vi "Apply Scaling Factor.vi"(6 "Apply to Vertex?":bool, 9 "Plot Representation Cluster":T3, 11 "2D Plot.lvclass in":refnum<class "2D Plot.lvclass">) -> (1 "Base Cluster":T2, 2 "Vertex Cluster":T1, 3 "2D Plot.lvclass out":refnum<class "2D Plot.lvclass">)   [LabVIEW 2020, in "2D Plot.lvclass"]
uses:
  <vilib>/Math Plots/2D Math Plots/2D Plot/2D Plot/2D Plot.lvclass
  <vilib>/Math Plots/2D Math Plots/2D Plot/2D Plot/Typedef/Plot Representation.ctl
  <vilib>/Math Plots/2D Math Plots/2D Plot/2D Plot/Typedef/Range Cluster.ctl
  <vilib>/Math Plots/2D Math Plots/2D Plot/2D Plot/2D Plot.lvclass/2D Plot.ctl
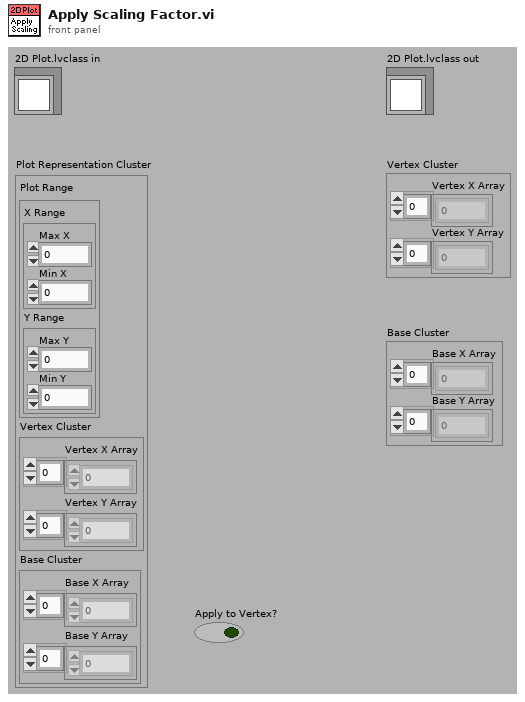
[diagram p1: front panel]
types:
  T1 = cluster{"Vertex X Array":dbl[], "Vertex Y Array":dbl[]}
  T2 = cluster{"Base X Array":dbl[], "Base Y Array":dbl[]}
  T3 = typedef "2D Plot.lvclass/Plot Representation.ctl" = cluster{"Plot Range":T4, "Vertex Cluster":cluster{"Vertex X Array":dbl[], "Vertex Y Array":dbl[]}, "Base Cluster":cluster{"Base X Array":dbl[], "Base Y Array":dbl[]}}
  T4 = typedef "2D Plot.lvclass/Range Cluster.ctl" = cluster{"X Range":cluster{"Max X":dbl, "Min X":dbl}, "Y Range":cluster{"Max Y":dbl, "Min Y":dbl}}
  T5 = typedef "2D Plot.lvclass/Scale Array.ctl" = T6[]
  T6 = typedef "2D Plot.lvclass/Scale Cluster.ctl" = cluster{"General":cluster{"Editable":bool, "Flipped":bool, "Mapping Mode":u8, "Visible":bool, "Style":u8, "Scale Fit":u8}, "Offset and Multiplier":T7, "Range":cluster{"Minimum":dbl, "Maximum":dbl, "Increment":dbl, "Minor Increment":dbl, "Start":dbl}, "Tick Color":cluster{"Major Color":u32, "Minor Color":u32}, "Gird Color":cluster{"Major Color":u32, "Minor Color":u32}, "Marker":cluster{"Visible":bool, "FG Color":u32, "BG Color":u32, "Font Name":string, "Font Size":u32, "Font Bold":bool, "Font Italic":bool, "Font Strikeout":bool, "Font Underline":bool}, "Name Label":cluster{"Visible":bool, "FG Color":u32, "BG Color":u32, "Font Name":string, "Font Size":u32, "Font Bold":bool, "Font Italic":bool, "Font Strikeout":bool, "Font Underline":bool, "Justification":enum16{"Left", "Center", "Right"}, "Text":string}}
  T7 = typedef "LVOffsetAndMultiplierTypeDef.ctl" = cluster{"Offset":dbl, "Multiplier":dbl}
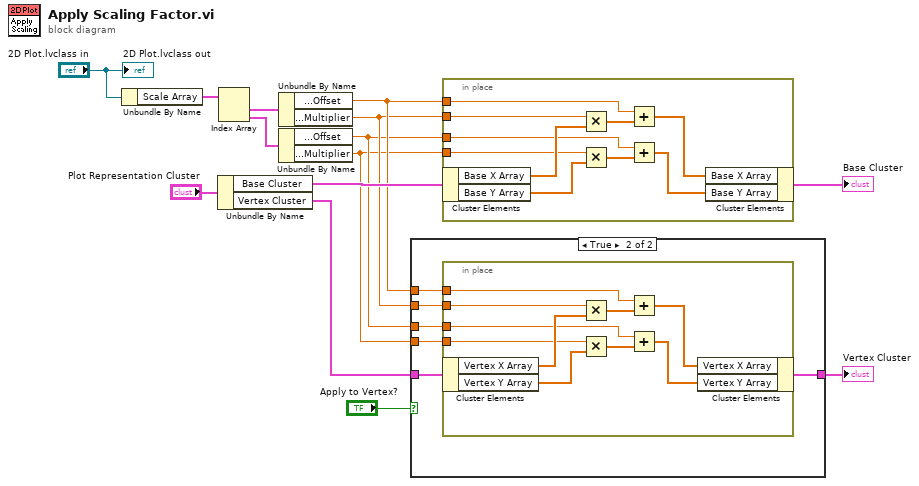
[diagram p0: block diagram]
diagram:
  n1 = Unbundle By Name("2D Plot.lvclass in") -> ("Scale Array"=w13:T5)
  n2 = Unbundle By Name("Plot Representation Cluster") -> ("Base Cluster"=w10:T2, "Vertex Cluster"=w3:T1)
  n3 = Index Array(array=w13) -> (element #1=w12:T6, element #2=w11:T6)  [unwired: 2 in]
  n4 = Unbundle By Name(w12) -> ("Offset and Multiplier.Offset"=w7:dbl, "Offset and Multiplier.Multiplier"=w6:dbl)
  n5 = Unbundle By Name(w11) -> ("Offset and Multiplier.Offset"=w5:dbl, "Offset and Multiplier.Multiplier"=w4:dbl)
  n6 = case shown="True" "Apply to Vertex?" {
    tunnel: w7 -> [_ w21]
    tunnel: w6 -> [_ w20]
    tunnel: w5 -> [_ w19]
    tunnel: w4 -> [_ w18]
    tunnel: w3 -> [w15 w17]
    tunnel: [w15 w16] -> w2
    frame False {
    }
    frame True {
      n7 = in-place {
        in-place-border: w20 -> [w23]
        in-place-border: w21 -> [w25]
        in-place-border: w18 -> [w22]
        in-place-border: w19 -> [w24]
        n8 = in-place-cluster #1(w17) -> ("Vertex X Array"=w29:dbl[], "Vertex Y Array"=w28:dbl[])
        n9 = Multiply(x=w23, y=w29) -> (x*y=w30:dbl[])
        n10 = Multiply(x=w22, y=w28) -> (x*y=w31:dbl[])
        n11 = Add(x=w25, y=w30) -> (x+y=w26:dbl[])
        n12 = Add(x=w24, y=w31) -> (x+y=w27:dbl[])
        n13 = in-place-cluster #1("Vertex X Array"=w26, "Vertex Y Array"=w27) -> (w16:T1)
      }
    }
  }
  "Vertex Cluster" <- w2
  n14 = in-place {
    in-place-border: w6 -> [w33]
    in-place-border: w7 -> [w35]
    in-place-border: w4 -> [w32]
    in-place-border: w5 -> [w34]
    n15 = in-place-cluster #2(w10) -> ("Base X Array"=w40:dbl[], "Base Y Array"=w37:dbl[])
    n16 = Multiply(x=w33, y=w40) -> (x*y=w41:dbl[])
    n17 = Multiply(x=w32, y=w37) -> (x*y=w38:dbl[])
    n18 = Add(x=w35, y=w41) -> (x+y=w39:dbl[])
    n19 = Add(x=w34, y=w38) -> (x+y=w36:dbl[])
    n20 = in-place-cluster #2("Base X Array"=w39, "Base Y Array"=w36) -> (→"Base Cluster":T2)
  }
  "2D Plot.lvclass out" <- "2D Plot.lvclass in"
